vi "Status Log FGV.vi"(7 "Action":T1=enum."Show Status File", 8 "error in":errorcluster, 10 "Status":string) -> (0 "error out":errorcluster)   [LabVIEW 2015]
doc: "let to open current status log file in the Windows NotePad"
uses:
  Status Log.ctl
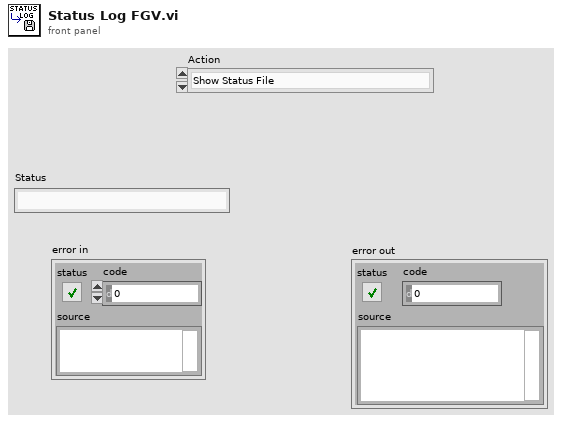
[diagram p1: front panel]
types:
  T1 = typedef "Status Log.ctl" = enum16{"Close file", "Open Status file", "Add Status", "Show Status File"}
  T2 = enum16{"open", "replace", "create", "open or create", "replace or create", "replace or create with confirmation"}
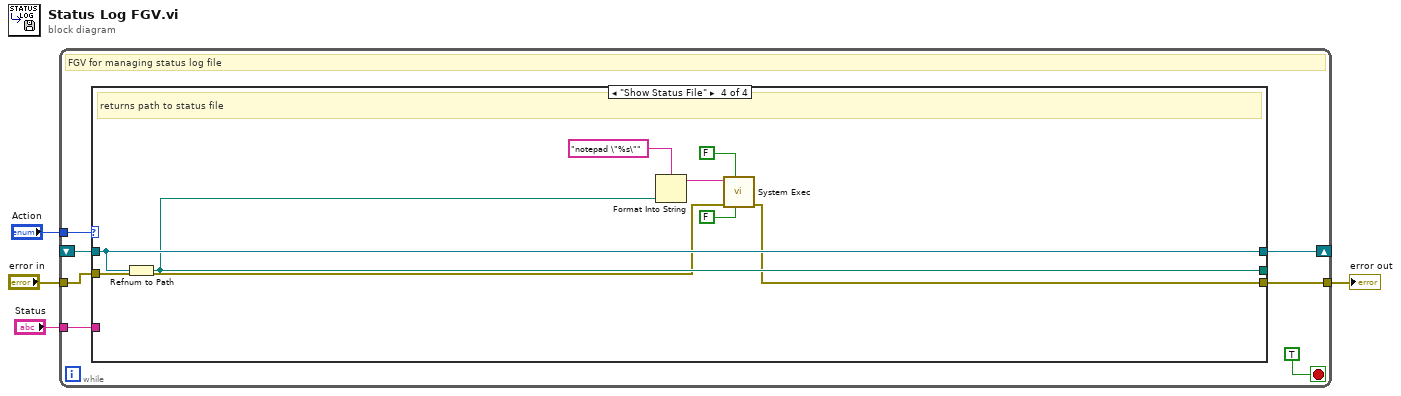
[diagram p0: block diagram]
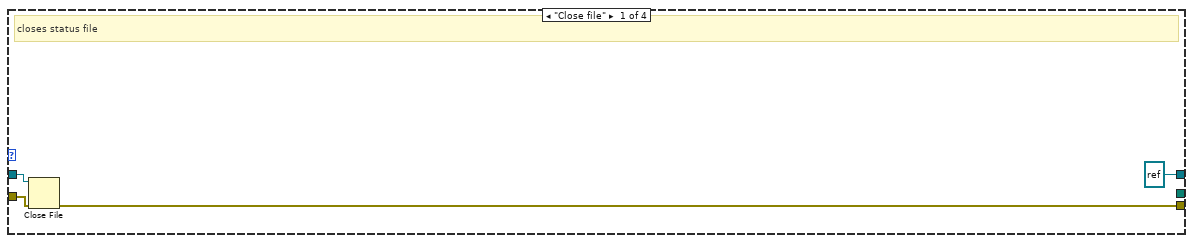
[diagram p2: hidden frame]
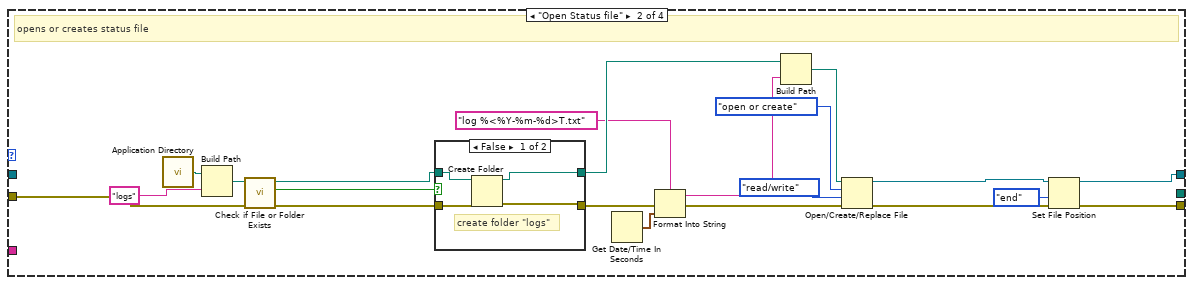
[diagram p3: hidden frame]
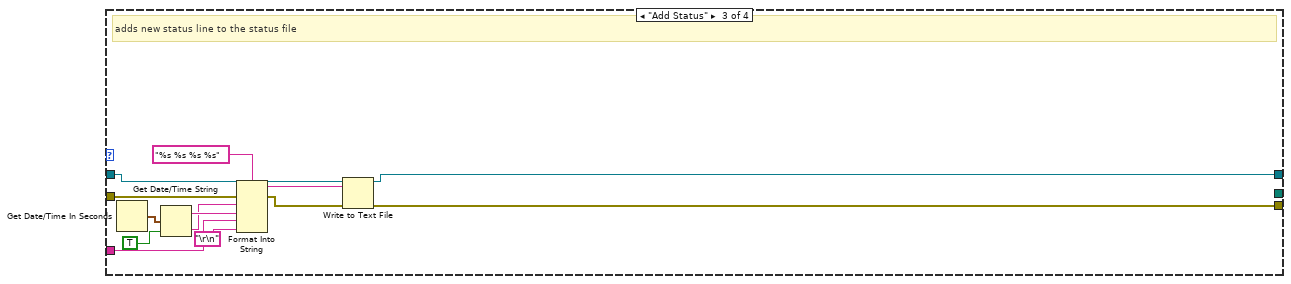
[diagram p5: hidden frame]
diagram:
  n1 = while {
    tunnel: "Action" -> [w10]
    tunnel: "Status" -> [w9]
    tunnel: [w8] -> w2
    tunnel: "error in" -> [w7]
    shift-right: [w5] -> _
    shift-left: _ -> [w6]
    stop <- TRUE stop-if-true
    # "FGV for managing status log file"
    n2 = case shown="\"Show Status File\"" w10 {
      tunnel: w9 -> [_ _ w49 _]
      tunnel: [w14 w28 w55 w59] -> w8
      tunnel: w7 -> [w15 w21 w46 w60]
      tunnel: [refnum<file> refnum ("refnum out") w27 w54 w63] -> w5
      tunnel: w6 -> [w13 _ w53 w63]
      tunnel: [_ _ _ w61] -> _
      frame "Close file" {
        # "closes status file"
        n3 = Close File(refnum=w13, error in=w15) -> (error out=w14:errorcluster)  [unwired: 1 out]
      }
      frame "Open Status file" {
        # "opens or creates status file"
        n4 = call <vilib>:"Application Directory.vi"() -> ("Application Directory"=w36:path)
        n5 = Build Path(base path=w36, name or relative path="logs") -> (appended path=w26:path)
        n6 = call <vilib>:"Check if File or Folder Exists.vi"("error in (no error)"=w21, "path"=w26) -> ("error out"=w22:errorcluster, "file or folder exists?"=w25:bool, "dup path"=w24:path)  [unwired: 7 in]
        n7 = case shown="False" w25 {
          tunnel: w24 -> [w38 w42]
          tunnel: [w37 w42] -> w23
          tunnel: w22 -> [w40 w41]
          tunnel: [w39 w41] -> w20
          frame False {
            # "create folder \"logs\""
            n8 = Create Folder(path (use dialog)=w38, error in=w40) -> (created path=w37:path, error out=w39:errorcluster)  [unwired: 1 in, 1 out]
          }
          frame True {
          }
        }
        n9 = Get Date/Time In Seconds() -> (seconds since 1Jan1904=w35:timestamp)
        n10 = Format Into String "Format Into String"(format string="log %<%Y-%m-%d>T.txt", error in=w20, w35) -> (resulting string=w33:string, error out=w34:errorcluster)  [unwired: 1 in]
        n11 = Build Path(base path=w23, name or relative path=w33) -> (appended path=w32:path)
        n12 = Open/Create/Replace File(file path (use dialog)=w32, error in=w34, operation (0:open)=T2."open or create", access (0:read/write)=enum16{"read/write", "read-only", "write-only"}."read/write") -> (refnum out=w29:refnum<file>, error out=w30:errorcluster)  [unwired: 2 in, 1 out]
        n13 = Set File Position(refnum=w29, from (0:start)=enum16{"start", "end", "current"}."end", error in=w30) -> (refnum out=w27:refnum<file>, error out=w28:errorcluster)  [unwired: 1 in]
      }
      frame "Add Status" {
        # "adds new status line to the status file"
        n14 = Get Date/Time In Seconds() -> (seconds since 1Jan1904=w43:timestamp)
        n15 = Get Date/Time String(seconds (now)=w43, want seconds? (F)=TRUE) -> (date string=w47:string, time string=w45:string)  [unwired: 1 in]
        n16 = Format Into String(format string="%s %s %s %s", error in=w46, w45, w47, w49, "\r\n") -> (resulting string=w51:string, error out=w52:errorcluster)  [unwired: 1 in]
        n17 = Write to Text File(file (use dialog)=w53, text=w51, error in=w52) -> (refnum out=w54:refnum<file>, error out=w55:errorcluster)  [unwired: 1 in, 1 out]
      }
      frame "Show Status File" {
        # "returns path to status file"
        n18 = Refnum to Path(1:w63) -> (0:w61:path)
        n19 = Format Into String(format string="notepad \"%s\"", w61) -> (resulting string=w62:string)  [unwired: 2 in, 1 out]
        n20 = call <vilib>:"System Exec.vi"("run minimized? (F)"=FALSE, "wait until completion? (T)"=FALSE, "error in (no error)"=w60, "command line"=w62) -> ("error out"=w59:errorcluster)  [unwired: 4 in, 3 out]
      }
    }
  }
  "error out" <- w2
